vi "T564_PolarityFromSETresponse.vi"(11 "String":string) -> (3 "Polarity":T1)   [LabVIEW 2013]
uses:
  ChannelPolarity.ctl
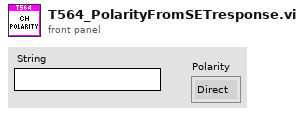
[diagram p1: front panel]
types:
  T1 = typedef "ChannelPolarity.ctl" = enum16{"Direct", "Inverted"}
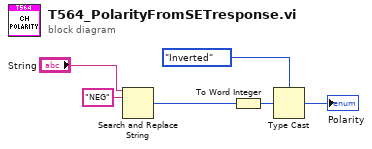
[diagram p0: block diagram]
diagram:
  n1 = Search and Replace String(input string="String", search string="NEG") -> (number of replacements=w1:i32)  [unwired: 6 in, 3 out]
  n2 = To Word Integer(number=w1) -> (16bit integer=w5:i16)
  n3 = Type Cast(type=ChannelPolarity."Inverted" ("Polarity"), x=w5) -> (*(type *) &x=→"Polarity":T1)
